vi "KH7008 Build Self Extracting Installer.vi"(8 "Path to project":path=path "C:/Users/ansom/Documents/GitHub/Krohn-Hite-7008/Krohn-Hite-7008 (x86).lvproj", 9 "Package Version":string="2.1.0.10") -> (0 "Error Out":errorcluster)   [LabVIEW 2019]
uses:
  <userlib>/LevyLab/Build Support/PostBuildSupport/PostBuildSupport.lvclass
  <userlib>/LevyLab/Build Support/Build/Build.lvlib
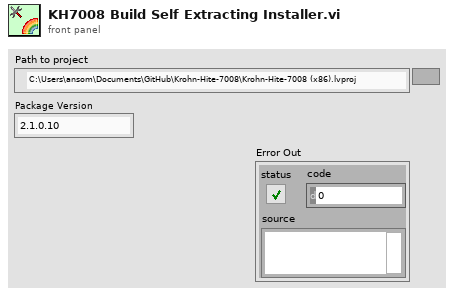
[diagram p1: front panel]
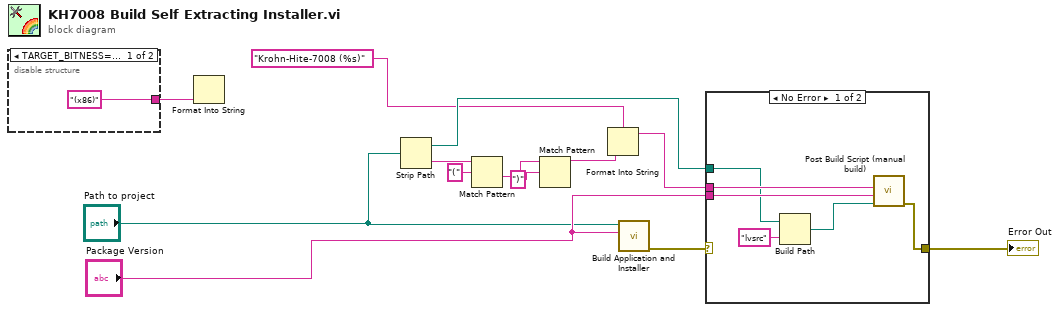
[diagram p0: block diagram]
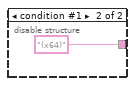
[diagram p3: hidden frame]
diagram:
  n1 = disable-structure shown="TARGET_BITNESS==32, Default" {
    disable-tunnel: ["(x86)" ("Name of build specification") "(x64)" ("Name of build specification")] -> w13
    frame condition #0 (active) {
    }
    frame condition #1 {
    }
  }
  n2 = Format Into String(w13) -> ()  [unwired: 3 in, 2 out]
  n3 = Strip Path(path="Path to project") -> (stripped path=w7:path, name=w12:string)
  n4 = Match Pattern(string=w12, regular expression="(") -> (after substring=w10:string)  [unwired: 1 in, 3 out]
  n5 = Match Pattern(string=w10, regular expression=")") -> (before substring=w8:string)  [unwired: 1 in, 3 out]
  n6 = Format Into String(format string="Krohn-Hite-7008 (%s)" ("Product Name"), w8) -> (resulting string=w5:string)  [unwired: 2 in, 1 out]
  n7 = call <userlib>:"Build Application and Installer.vi"("Package Version"="Package Version", "Path to project"="Path to project") -> ("error out"=w6:errorcluster)  [unwired: 9 in]
  n8 = case shown="No Error" w6 {
    selector: w6 -> [_ w22]
    tunnel: w5 -> [w21 _]
    tunnel: "Package Version" -> [w20 _]
    tunnel: w7 -> [w17 _]
    tunnel: [w16 w22] -> w1
    frame No Error {
      n9 = Build Path(base path=w17, name or relative path="lvsrc") -> (appended path=w18:path)
      n10 = call <userlib>:"Post Build Script (manual build).vi"("Package Source Folder"=w18, "Package Version"=w20, "Product Name"=w21) -> ("error out"=w16:errorcluster)  [unwired: 8 in]
    }
    frame Error {
    }
  }
  "Error Out" <- w1
